vi "DSF.Engine.Framework.Initialize Engine Channels Base Pointer.vi"(8 "error in (no error)":errorcluster, 10 "Engine Channels Pointer":refnum<class "DSF.Engine.Pointer.DBL.lvclass">, 11 "Framework in":refnum<class "DSF.Engine.Framework.lvclass">) -> (0 "error out":errorcluster, 3 "Framework out":refnum<class "DSF.Engine.Framework.lvclass">)   [LabVIEW 2017, in "DSF.Engine.lvlib" / "DSF.Engine.Framework.lvclass"]
uses:
  DSF.Engine.Framework.lvclass
  Pointer/DSF.Engine.Pointer.DBL.lvclass
  DSF.Engine.Framework.lvclass/DSF.Engine.Framework.ctl
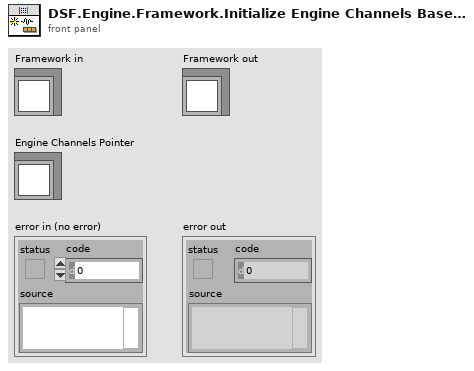
[diagram p1: front panel]
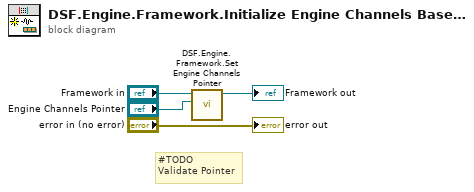
[diagram p0: block diagram]
diagram:
  # "#TODO\nValidate Pointer"
  n1 = call "DSF.Engine.Framework.Set Engine Channels Pointer.vi"("Engine Channels Pointer"="Engine Channels Pointer", "Framework in"="Framework in") -> ("Framework out"=→"Framework out":refnum<class "DSF.Engine.Framework.lvclass">)  [unwired: 9 in]
  "error out" <- "error in (no error)"
